vi "MemCopy.vi"(8 "error in (no error)":errorcluster, 10 "LIMPICTURE in":T1, 11 "hFile in":T2) -> (0 "error out":errorcluster, 1 "pBuffer out":u8[](array[numeric]), 2 "LIMPICTURE out":T1, 3 "hFile out":T2)   [LabVIEW 2014, in "ND2_Reader_32.lvlib"]
doc: "This uses Built In DLL routine (memcpy) to copy data from ND2 Data Space to something LabVIEW can use"
uses:
  ND2_Reader_32.lvlib
  controls/numeric_LIMFILEHANDLE.ctl
  controls/cluster_LIMPICTURE.ctl
  <vilib>/Utility/sysdir.llb/System Directory Type.ctl
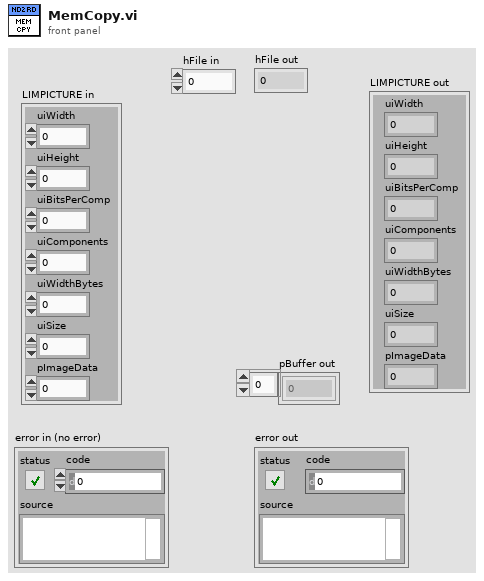
[diagram p1: front panel]
types:
  T1 = typedef "cluster_LIMPICTURE.ctl" = cluster{"uiWidth":u32, "uiHeight":u32, "uiBitsPerComp":u32, "uiComponents":u32, "uiWidthBytes":u32, "uiSize":u32, "pImageData":u32}
  T2 = typedef "numeric_LIMFILEHANDLE.ctl" = i32
  T3 = typedef "System Directory Type.ctl" = i32
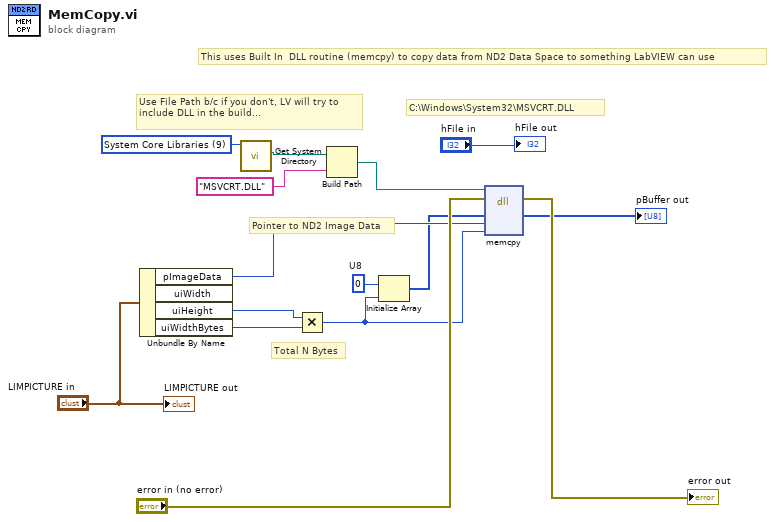
[diagram p0: block diagram]
diagram:
  w5 = T3 9 items=["User Home"=0, "User Desktop"=1, "User Documents"=2, "User Application Data"=3, "User Preferences"=4, "User Temporary"=5, "Public Documents"=6, "Public Application Data"=7, "Public Preferences"=8, "Public Cache"=13, "System Core Libraries"=9, "System Installed Libraries"=10, "Application Files"=11, "Boot Volume Root"=12] ("system directory type")
  w13 = u8 0  # U8
  # "Use File Path b/c if you don't, LV will try to include DLL in the build..."
  # "This uses Built In  DLL routine (memcpy) to copy data from ND2 Data Space to something LabVIEW can use"
  # "Total N Bytes"
  # "Pointer to ND2 Image Data"
  # "C:\\Windows\\System32\\MSVCRT.DLL"
  n1 = Unbundle By Name("LIMPICTURE in") -> ("pImageData"=w8:u32, "uiHeight"=w11:u32, "uiWidthBytes"=w12:u32)  [unwired: 1 out]
  n2 = call <vilib>:"Get System Directory.vi"("system directory type"=w5) -> ("system directory"=w4:path)  [unwired: 10 in]
  n3 = Multiply(x=w11, y=w12) -> (x*y=w10:u32)
  n4 = Build Path(base path=w4, name or relative path="MSVCRT.DLL") -> (appended path=w2:path)
  n5 = Initialize Array(w13, w10) -> (w7:u8[])
  n6 = dll-call lib="C:/Windows/System32/MSVCRT.DLL" fn="memcpy"(path in=w2, error in="error in (no error)", "dest"=w7, "source"=w8, "buffsize"=w10) -> (error out=→"error out":errorcluster, "dest"=→"pBuffer out":u8[])  [unwired: 1 in, 4 out]
  "hFile out" <- "hFile in"
  "LIMPICTURE out" <- "LIMPICTURE in"
